vi "MWP.vi"(11 "Numeric":dbl) -> (3 "³t¤ñ":dbl[](array[numeric]))   [LabVIEW 2019]
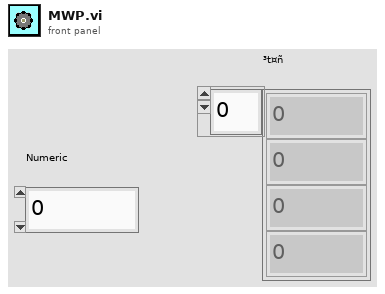
[diagram p1: front panel]
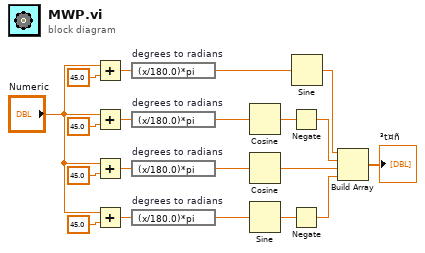
[diagram p0: block diagram]
diagram:
  n1 = Add(x="Numeric", y=45.0) -> (x+y=w16:dbl)
  n2 = Add(x="Numeric", y=45.0) -> (x+y=w6:dbl)
  n3 = Add(x="Numeric", y=45.0) -> (x+y=w13:dbl)
  n4 = Add(x="Numeric", y=45.0) -> (x+y=w7:dbl)
  n5 = expression code="(x/180.0)*pi" "degrees to radians"(w16) -> (w20:dbl)
  n6 = expression code="(x/180.0)*pi" "degrees to radians"(w6) -> (w19:dbl)
  n7 = expression code="(x/180.0)*pi" "degrees to radians"(w13) -> (w12:dbl)
  n8 = expression code="(x/180.0)*pi" "degrees to radians"(w7) -> (w10:dbl)
  n9 = Cosine(x=w19) -> (cos(x)=w5:dbl)
  n10 = Cosine(x=w12) -> (cos(x)=w11:dbl)
  n11 = Sine(x=w10) -> (sin(x)=w2:dbl)
  n12 = Negate(x=w5) -> (-x=w4:dbl)
  n13 = Negate(x=w2) -> (-x=w3:dbl)
  n14 = Sine(x=w20) -> (sin(x)=w18:dbl)
  n15 = Build Array(w18, w4, w11, w3) -> (→"³t¤ñ":dbl[])
